vi "Configure Device.vi"(8 "error in":errorcluster, 11 "PPT in":refnum<class "PPT.lvclass">) -> (0 "error out":errorcluster, 3 "PPT out":refnum<class "PPT.lvclass">, 4 "SP":dbl, 5 "Settable?":bool)   [LabVIEW 2014, in "PPT Library.lvlib" / "PPT.lvclass"]
uses:
  PPT.lvclass
  reusable/Session APIs/Serial/Serial Session.lvclass
  Configurable Device/Configurable Device.lvclass/Configurable Device.ctl
  PPT.lvclass/PPT.ctl
  reusable/Session APIs/File Access/Config Data/Config Data.lvclass/Config Data.ctl
  Configurable Device/Read Handle.vi
  Configurable Device/Accessors/Write type.vi
  Configurable Device/Accessors/Write controller_.vi
  Accessors/Write Serial Session.vi
  Configurable Device/Read ID.vi
  reusable/Session APIs/File Access/Config Data/Accessors/Read Ref.vi
  Accessors/Write Address.vi
  Configurable Device/Read Log Session.vi
  Configurable Device/Accessors/Write Addr.vi
  Configurable Device/Accessors/Write Model.vi
  Configurable Device/Accessors/Write label.vi
  <vilib>/Utility/config.llb/Read Key (U32).vi
  <vilib>/Utility/config.llb/Read Key (String).vi
  Configurable Device/Configurable Device.lvclass
  reusable/Session APIs/File Access/Config Data/Config Data.lvclass
  <userlib>/_Session Fwk/Session - Root.lvclass
  <vilib>/ErrorRing/Error Ring.xnode
  <vilib>/Utility/config.llb/NI_LVConfig.lvlib
  reusable/Session APIs/Session Log/System Log.lvclass
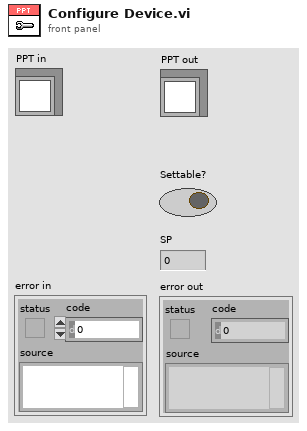
[diagram p1: front panel]
types:
  T1 = enum16{"atm", "bar", "cmwc", "ftwc", "inhg", "inwc", "kgcm", "kpa", "mbar", "mmhg", "mpa", "mwc", "psi", "user", "lcom", "pfs"}
  T2 = typedef "Serial Session.lvclass/Session Handle.ctl" = refnum<data-value>
  T3 = typedef "Config Data.lvclass/Config Session.ctl" = refnum<data-value>
  T4 = typedef "NI_LVConfig.lvlib/Config Data RefNum.ctl" = refnum<k1>
  T5 = typedef "Session - Root.lvclass/Session Handle.ctl" = refnum<data-value>
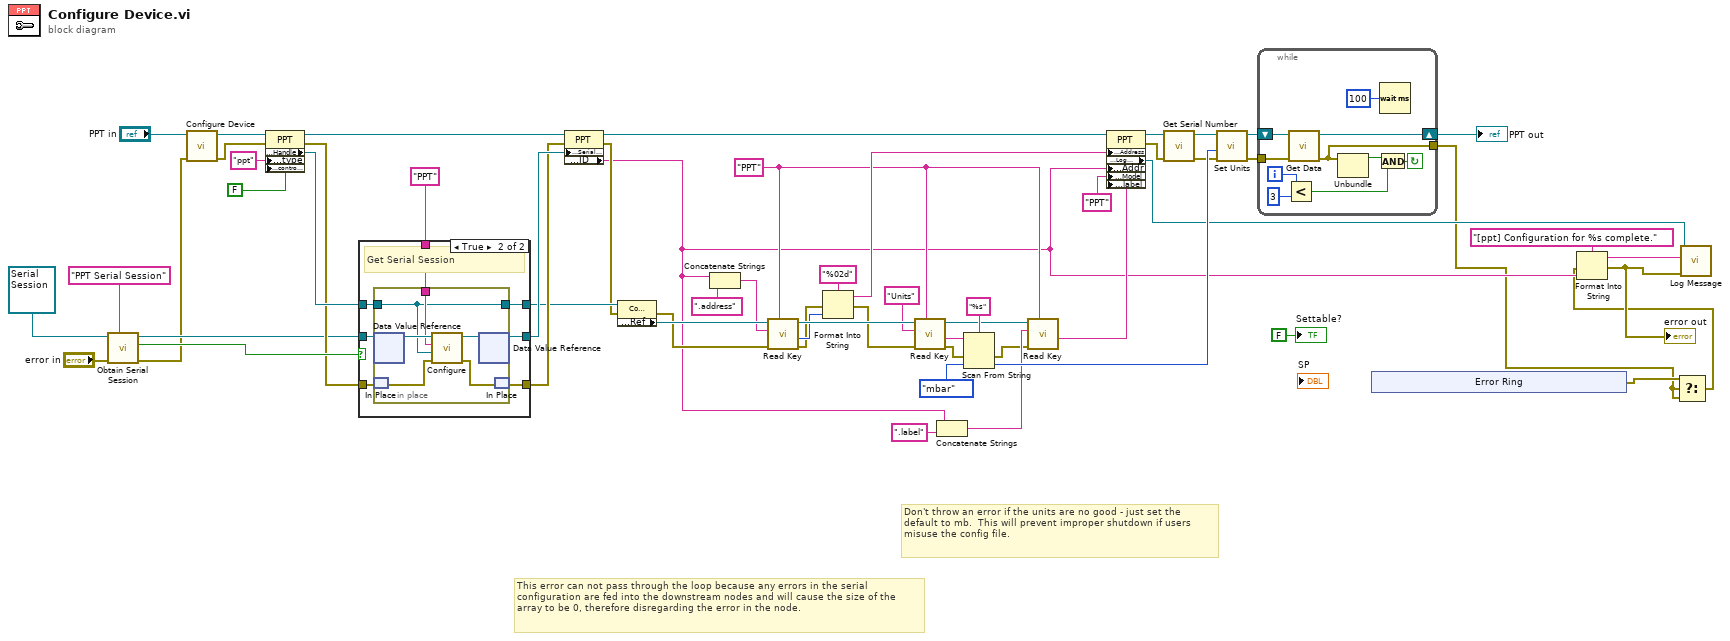
[diagram p0: block diagram]
diagram:
  w9 = "PPT" ("section")
  # "This error can not pass through the loop because any errors in the serial configuration are fed into the downstream nodes and will cause the size of the array to be 0, therefore disregarding the error in the node."
  # "Don't throw an error if the units are no good - just set the default to mb.  This will prevent improper shutdown if users misuse the config file."
  n1 = call "Obtain Serial Session.vi"("Session Name ()"="PPT Serial Session", "error in"="error in", "Serial Session in"=refnum<class "Serial Session.lvclass"> refnum) -> ("error out"=w14:errorcluster, "created new?"=w59:bool, "hSerial"=w55:T2)  [unwired: 6 in]
  n2 = call-parent "Configure Device.vi"("error in"=w14, "Device in"="PPT in") -> ("error out"=w13:errorcluster, "Device out"=w15:refnum<class "PPT.lvclass">)  [unwired: 6 in, 2 out]
  n3 = property class="PPT"(reference=w15, error in=w13, "Accessors:type"="ppt" ("type"), "Accessors:controller_"=FALSE ("controller_")) -> (reference out=w51:refnum<class "PPT.lvclass">, error out=w57:errorcluster, "Accessors:Handle"=w58:T3)
  n4 = case shown="True" w59 {
    tunnel: w55 -> [w62 w69]
    tunnel: w57 -> [w61 w65]
    tunnel: [w62 w68] -> w50
    tunnel: [w61 w67] -> w49
    tunnel: w58 -> [w60 w66]
    tunnel: [w60 w64] -> w40
    tunnel: "PPT" ("section") -> [_ w63]
    frame False {
    }
    frame True {
      # "Get Serial Session"
      n5 = in-place {
        in-place-border: w66 -> [w70]
        in-place-border: w63 -> [w71]
        in-place-border: [w70] -> w64
        n6 = in-place-dvr #1(w69) -> (w75:refnum<class "Serial Session.lvclass">)  [unwired: 1 out]
        n7 = in-place-match #2(w65) -> (w74:errorcluster)
        n8 = call "Configure.vi"("error in"=w74, "Config Handle"=w70, "section"=w71, "Serial Session in"=w75) -> ("error out"=w73:errorcluster, "Serial Session out"=w72:refnum<class "Serial Session.lvclass">)  [unwired: 6 in]
        n9 = in-place-dvr #1(w72) -> (w68:T2)  [unwired: 1 out]
        n10 = in-place-match #2(w73) -> (w67:errorcluster)
      }
    }
  }
  n11 = property class="PPT"(reference=w51, error in=w49, "Accessors:Serial Session"=w50) -> (reference out=w46:refnum<class "PPT.lvclass">, error out=w39:errorcluster, "Accessors:ID"=w5:string)
  n12 = property class="Config Data"(reference=w40, error in=w39) -> (error out=w27:errorcluster, "Accessors:Ref"=w38:T4)  [unwired: 1 out]
  n13 = Concatenate Strings(w5, ".address" ("string")) -> (w8:string)
  n14 = call-poly <vilib>:"Read Key.vi"("section"=w9, "error in (no error)"=w27, "key"=w8, "refnum"=w38) -> ("error out"=w26:errorcluster, "value"=w36:u32, "refnum out"=w48:T4)  [unwired: 4 in, 1 out]
  n15 = Format Into String(format string="%02d", error in=w26, w36) -> (resulting string=w45:string, error out=w25:errorcluster)  [unwired: 1 in]
  n16 = call-poly <vilib>:"Read Key.vi"("section"=w9, "error in (no error)"=w25, "key"="Units", "refnum"=w48) -> ("error out"=w31:errorcluster, "value"=w44:string, "refnum out"=w10:T4)  [unwired: 4 in, 1 out]
  n17 = Concatenate Strings(w5, ".label" ("string")) -> (w11:string)
  n18 = Scan From String(format string="%s", input string=w44, error in=w31, default 1=T1."mbar" ("units")) -> (error out=w6:errorcluster, output 1=w41:T1)  [unwired: 1 in, 2 out]
  n19 = call-poly <vilib>:"Read Key.vi"("section"=w9, "error in (no error)"=w6, "key"=w11, "refnum"=w10) -> ("value"=w7:string)  [unwired: 4 in, 3 out]
  n20 = property class="PPT"(reference=w46, "Accessors:Address"=w45, "Accessors:Addr"=w5, "Accessors:Model"="PPT" ("Model"), "Accessors:label"=w7) -> (reference out=w23:refnum<class "PPT.lvclass">, error out=w21:errorcluster, "Accessors:Log Session"=w34:T5)  [unwired: 1 in]
  n21 = call "Get Serial Number.vi"("error in"=w21, "PPT in"=w23) -> ("error out"=w20:errorcluster, "PPT out"=w22:refnum<class "PPT.lvclass">)  [unwired: 7 in, 1 out]
  n22 = call "Set Units.vi"("error in"=w20, "units"=w41, "PPT in"=w22) -> ("error out"=w28:errorcluster, "PPT out"=w30:refnum<class "PPT.lvclass">)  [unwired: 7 in]
  n23 = while {
    shift-right: [w84] -> w29
    shift-left: w30 -> [w85]
    tunnel: [w78] -> w2
    tunnel: w28 -> [w77]
    i -> [w82]
    stop <- w79 continue-if-true
    n24 = Less?(x=w82, y=3) -> (x < y?=w80:bool)
    n25 = call-dynamic "Get Data.vi"("error in"=w77, "PPT in"=w85) -> ("error out"=w78:errorcluster, "PPT out"=w84:refnum<class "PPT.lvclass">)  [unwired: 7 in, 1 out]
    n26 = Unbundle(w78) -> ("status"=w83:bool)  [unwired: 2 out]
    n27 = And(x=w83, y=w80) -> (x .and. y?=w79:bool)
    n28 = Wait (ms)(milliseconds to wait=u32 100) -> ()  [unwired: 1 out]
  }
  "PPT out" <- w29
  n29 = xnode "Error Ring"() -> ("error out"=w3:errorcluster)
  n30 = Select(t=w3, s=w2, f=w2) -> (s? t:f=w1:errorcluster)
  n31 = Format Into String(format string="[ppt] Configuration for %s complete.", error in=w1, w5) -> (resulting string=w32:string, error out=w4:errorcluster)  [unwired: 1 in]
  "error out" <- w4
  n32 = call "Log Message.vi"("error in"=w4, "MSG In"=w32, "session in"=w34) -> ()  [unwired: 7 in, 2 out]
  "Settable?" <- FALSE ("Settable?")
